vi "Include Build Assets.vi"(8 "error in":errorcluster, 11 "Project ref":refnum<vi>) -> (0 "error out":errorcluster)   [LabVIEW 2020, in "MeasurementService Editor.lvlib"]
uses:
  MeasurementService Editor.lvlib
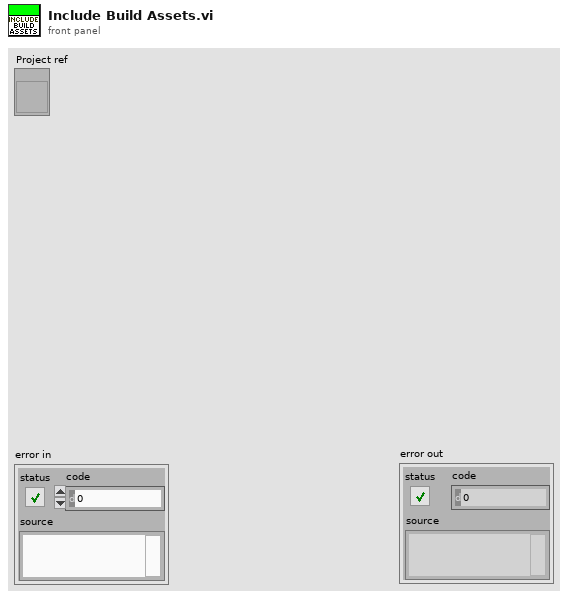
[diagram p1: front panel]
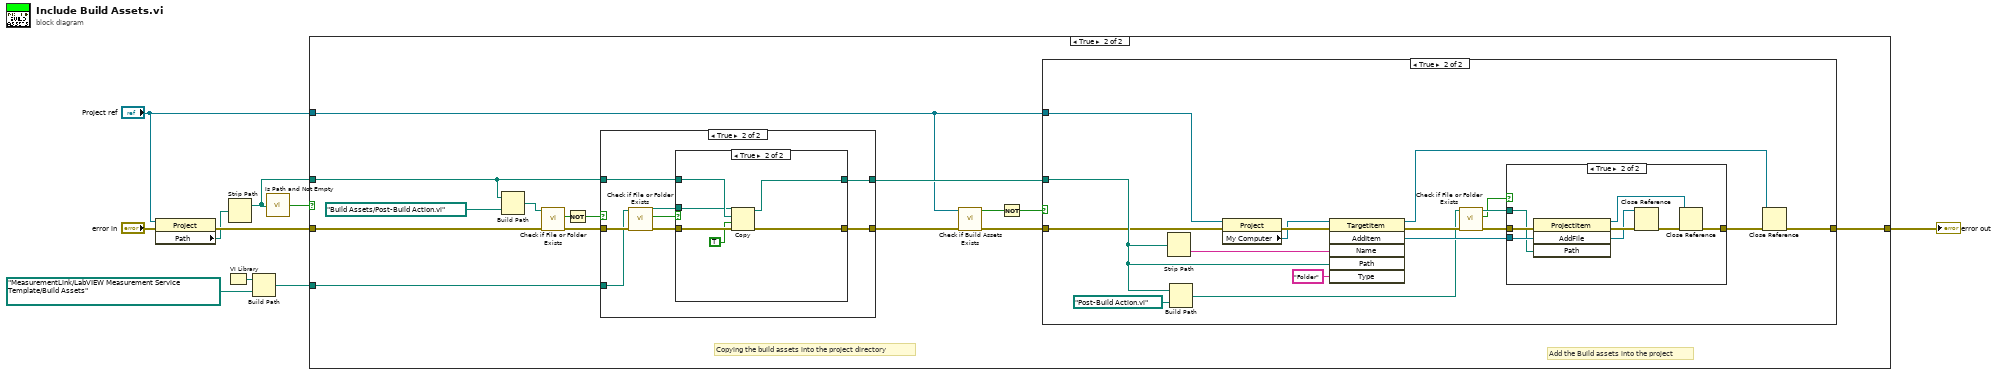
[diagram p0: block diagram]
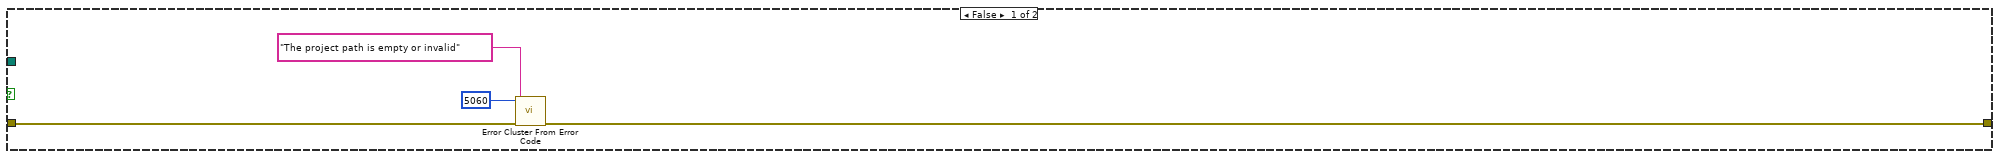
[diagram p2: hidden frame]
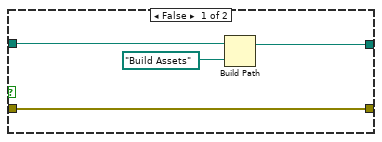
[diagram p3: hidden frame]
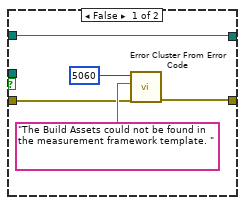
[diagram p4: hidden frame]
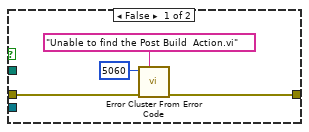
[diagram p6: hidden frame]
diagram:
  n1 = property class="Project"(reference="Project ref", error in="error in") -> (error out=w7:errorcluster, "Path"=w2:path)  [unwired: 1 out]
  n2 = VI Library() -> (path=w6:path)
  n3 = Strip Path(path=w2) -> (stripped path=w1:path)  [unwired: 1 out]
  n4 = Build Path(base path=w6, name or relative path=path "MeasurementLink/LabVIEW Measurement Service Template/Build Assets") -> (appended path=w4:path)
  n5 = call <vilib>:"Is Path and Not Empty.vi"("path"=w1) -> ("Is Path and Not Empty?"=w10:bool)  [unwired: 4 in]
  n6 = case shown="True" w10 {
    tunnel: w7 -> [w14 w29]
    tunnel: [w13 w28] -> w9
    tunnel: w4 -> [_ w20]
    tunnel: w1 -> [_ w22]
    tunnel: "Project ref" -> [_ w17]
    frame False {
      n7 = call <vilib>:"Error Cluster From Error Code.vi"("error in (no error)"=w14, "error message (\"\")"="The project path is empty or invalid" ("error message (\"\")"), "error code (0)"=5060) -> ("error out"=w13:errorcluster)  [unwired: 6 in]
    }
    frame True {
      # "Add the Build assets into the project"
      # "Copying the build assets into the project directory"
      n8 = Build Path(base path=w22, name or relative path=path "Build Assets/Post-Build Action.vi") -> (appended path=w26:path)
      n9 = call <vilib>:"Check if File or Folder Exists.vi"("error in (no error)"=w29, "path"=w26) -> ("error out"=w24:errorcluster, "file or folder exists?"=w25:bool)  [unwired: 7 in, 1 out]
      n10 = Not(x=w25) -> (.not. x?=w23:bool)
      n11 = case shown="True" w23 {
        tunnel: w24 -> [w30 w41]
        tunnel: [w30 w40] -> w19
        tunnel: w22 -> [w33 w39]
        tunnel: [w31 w38] -> w21
        tunnel: w20 -> [_ w36]
        frame False {
          n12 = Build Path(base path=w33, name or relative path=path "Build Assets") -> (appended path=w31:path)
        }
        frame True {
          n13 = call <vilib>:"Check if File or Folder Exists.vi"("error in (no error)"=w41, "path"=w36) -> ("error out"=w37:errorcluster, "file or folder exists?"=w35:bool, "dup path"=w34:path)  [unwired: 7 in]
          n14 = case shown="True" w35 {
            tunnel: w37 -> [w43 w52]
            tunnel: [w42 w51] -> w40
            tunnel: w39 -> [w46 w50]
            tunnel: [w46 w49] -> w38
            tunnel: w34 -> [_ w47]
            frame False {
              n15 = call <vilib>:"Error Cluster From Error Code.vi"("error in (no error)"=w43, "error message (\"\")"="The Build Assets could not be found in the measurement framework template. " ("error message (\"\")"), "error code (0)"=5060) -> ("error out"=w42:errorcluster)  [unwired: 6 in]
            }
            frame True {
              n16 = Copy(8:w52, 9:TRUE ("overwrite (F)"), 10:w50, 11:w47) -> (0:w51:errorcluster, 3:w49:path)  [unwired: 1 in, 1 out]
            }
          }
        }
      }
      n17 = call "Check if Build Assets Exists.vi"("error in"=w19, "Project ref"=w17) -> ("error out"=w18:errorcluster, "Build Assests exists?"=w16:bool)  [unwired: 8 in]
      n18 = Not(x=w16) -> (.not. x?=w15:bool)
      n19 = case shown="True" w15 {
        tunnel: [w53 w70] -> w28
        tunnel: w17 -> [_ w69]
        tunnel: w21 -> [_ w68]
        tunnel: w18 -> [w53 w67]
        frame False {
          # "Ignore the process since the project already contains the required files"
        }
        frame True {
          n20 = Strip Path(path=w68) -> (name=w62:string)  [unwired: 1 out]
          n21 = Build Path(base path=w68, name or relative path=path "Post-Build Action.vi") -> (appended path=w57:path)
          n22 = property class="Project"(reference=w69, error in=w67) -> (error out=w66:errorcluster, "My Computer"=w64:refnum<vi>)  [unwired: 1 out]
          n23 = invoke class="TargetItem" method="AddItem"(reference=w64, error in=w66, "Name"=w62, "Path"=w68, "Type"="Folder") -> (reference out=w63:refnum<vi>, error out=w65:errorcluster, "AddItem"=w60:refnum<vi>)  [unwired: 1 in, 3 out]
          n24 = call <vilib>:"Check if File or Folder Exists.vi"("error in (no error)"=w65, "path"=w57) -> ("error out"=w58:errorcluster, "file or folder exists?"=w55:bool, "dup path"=w56:path)  [unwired: 7 in]
          n25 = case shown="True" w55 {
            tunnel: w58 -> [w74 w82]
            tunnel: w60 -> [_ w81]
            tunnel: w56 -> [_ w80]
            tunnel: [w73 w75] -> w54
            frame False {
              n26 = call <vilib>:"Error Cluster From Error Code.vi"("error in (no error)"=w74, "error message (\"\")"="Unable to find the Post Build  Action.vi" ("error message (\"\")"), "error code (0)"=5060) -> ("error out"=w73:errorcluster)  [unwired: 6 in]
            }
            frame True {
              n27 = invoke class="ProjectItem" method="AddFile"(reference=w81, error in=w82, "Path"=w80) -> (reference out=w78:refnum<vi>, error out=w77:errorcluster, "AddFile"=w76:refnum<vi>)  [unwired: 1 in, 1 out]
              n28 = Close Reference(reference=w76, error in (no error)=w77) -> (error out=w79:errorcluster)
              n29 = Close Reference(reference=w78, error in (no error)=w79) -> (error out=w75:errorcluster)
            }
          }
          n30 = Close Reference(reference=w63, error in (no error)=w54) -> (error out=w70:errorcluster)
        }
      }
    }
  }
  "error out" <- w9
